vi "PulseTrain-Create.vi"(8 "error in (no error)":errorcluster, 9 "Npts":i32, 10 "Sampling Rate (Hz)":dbl, 11 "Pulse Train Params":T1) -> (0 "error out":errorcluster, 1 "Waveform":dbl[](array[numeric]), 2 "Sampling Rate (thru)":dbl, 3 "Pulse Train Params (out)":T1)   [LabVIEW 2020]
uses:
  Pulse Train Params.ctl
  Pulse Polarity.ctl
  PT-Continuous State.ctl
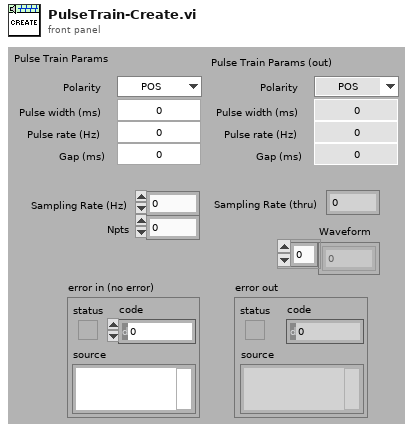
[diagram p1: front panel]
types:
  T1 = typedef "Pulse Train Params.ctl" = cluster{"Pulse width (us)":dbl, "Pulse rate (Hz)":dbl, "Gap (ms)":dbl, "Polarity":T2, "PT State":T3, "Asynch":bool}
  T2 = typedef "Pulse Polarity.ctl" = enum16{"POS", "NEG", "POS-NEG", "NEG-POS"}
  T3 = typedef "PT-Continuous State.ctl" = cluster{"Template":dbl[], "Nperiod":i32, "Index":i32, "Pulse Rate (Hz)":dbl, "Phase (cycles)":dbl, "Noff":i32}
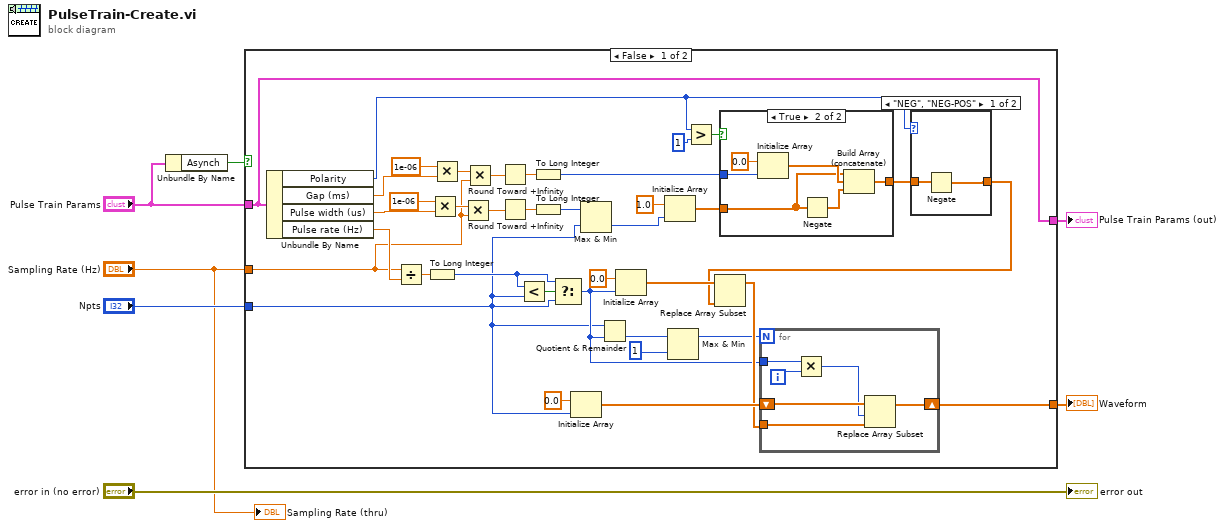
[diagram p0: block diagram]
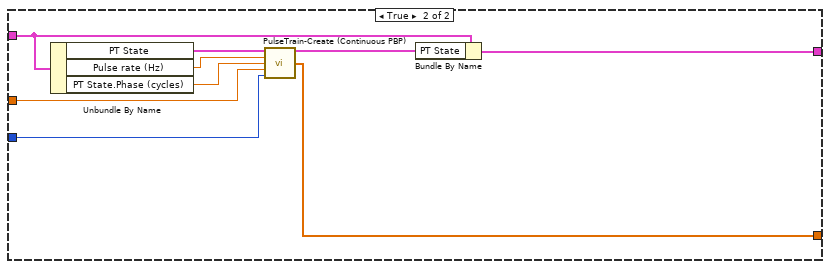
[diagram p4: hidden frame]
diagram:
  n1 = Unbundle By Name("Pulse Train Params") -> ("Asynch"=w2:bool)
  n2 = case shown="False" w2 {
    tunnel: "Npts" -> [w8 w65]
    tunnel: [w28 w64] -> w5
    tunnel: "Sampling Rate (Hz)" -> [w25 w66]
    tunnel: "Pulse Train Params" -> [w11 w63]
    tunnel: [w11 w61] -> w1
    frame False {
      n3 = Unbundle By Name(w11) -> ("Polarity"=w17:T2, "Gap (ms)"=w24:dbl, "Pulse width (us)"=w39:dbl, "Pulse rate (Hz)"=w44:dbl)
      n4 = Divide(x=w25, y=w44) -> (x/y=w43:dbl)
      n5 = To Long Integer(number=w43) -> (32bit integer=w41:i32)
      n6 = Multiply(x=1e-06, y=w39) -> (x*y=w37:dbl)
      n7 = Multiply(x=1e-06, y=w24) -> (x*y=w26:dbl)
      n8 = Multiply(x=w37, y=w25) -> (x*y=w36:dbl)
      n9 = Multiply(x=w26, y=w25) -> (x*y=w22:dbl)
      n10 = Round Toward +Infinity(x=w22) -> (ceil(x): smallest int >= x=w23:dbl)
      n11 = Round Toward +Infinity(x=w36) -> (ceil(x): smallest int >= x=w35:dbl)
      n12 = Less?(x=w41, y=w8) -> (x < y?=w42:bool)
      n13 = To Long Integer(number=w23) -> (32bit integer=w18:i32)
      n14 = To Long Integer(number=w35) -> (32bit integer=w10:i32)
      n15 = Select(t=w41, s=w42, f=w8) -> (s? t:f=w29:i32)
      n16 = Initialize Array(0.0 ("element"), w8) -> (w31:dbl[])
      n17 = Max & Min(x=w10, y=w8) -> (min(x,y)=w9:i32)  [unwired: 1 out]
      n18 = Quotient & Remainder(x=w8, y=w29) -> (floor(x/y)=w13:i32)  [unwired: 1 out]
      n19 = Initialize Array(0.0 ("element"), w29) -> (w40:dbl[])
      n20 = Initialize Array(1.0 ("element"), w9) -> (w19:dbl[])
      n21 = Max & Min(x=w13, y=1 ("x")) -> (max(x,y)=w14:i32)  [unwired: 1 out]
      n22 = Greater?(x=w17, y=u16 1) -> (0:w21:bool)
      n23 = case shown="True" w21 {
        tunnel: w19 -> [w48 w51]
        tunnel: w18 -> [_ w54]
        tunnel: [w48 w49] -> w16
        frame False {
        }
        frame True {
          n24 = Initialize Array(0.0 ("element"), w54) -> (w52:dbl[])
          n25 = Negate(x=w51) -> (-x=w50:dbl[])
          n26 = Build Array (concatenate)(w51, w52, w50) -> (w49:dbl[])
        }
      }
      n27 = case shown="\"NEG\", \"NEG-POS\"" w17 {
        tunnel: w16 -> [w46 w47]
        tunnel: [w45 w47] -> w15
        frame "NEG", "NEG-POS" {
          n28 = Negate(x=w46) -> (-x=w45:dbl[])
        }
        frame "POS", "POS-NEG", Default {
        }
      }
      n29 = Replace Array Subset(array=w40, new element=w15) -> (w30:dbl[])  [unwired: 1 in]
      n30 = for {
        N: w14 -> [_]
        tunnel: w30 -> [w58]
        shift-right: [w59] -> w28
        shift-left: w31 -> [w60]
        tunnel: w29 -> [w57]
        i -> [w56]
        n31 = Multiply(x=w57, y=w56) -> (x*y=w55:i32)
        n32 = Replace Array Subset(array=w60, new element=w58, index=w55) -> (w59:dbl[])
      }
    }
    frame True {
      n33 = Unbundle By Name(w63) -> ("PT State"=w69:T3, "Pulse rate (Hz)"=w68:dbl, "PT State.Phase (cycles)"=w67:dbl)
      n34 = call "PulseTrain-Create (Continuous PBP).vi"("State In"=w69, "Pulse Rate (Hz)"=w68, "Phase (cycles)"=w67, "Fs (Hz)"=w66, "Npts"=w65) -> ("State Out"=w62:T3, "Buffer"=w64:dbl[])  [unwired: 8 in, 1 out]
      n35 = Bundle By Name(cluster=w63, "PT State"=w62) -> (w61:T1)
    }
  }
  "Waveform" <- w5
  "Pulse Train Params (out)" <- w1
  "error out" <- "error in (no error)"
  "Sampling Rate (thru)" <- "Sampling Rate (Hz)"
